vi "GenerateLog.vi"() -> (2 "JSON":string, 3 "MsgCluster":T1)   [LabVIEW 2020, in "ORM_Examples.lvlib" / "syslogs.lvclass"]
uses:
  syslogs.lvclass
  SysLogLog_cluster.ctl
  <vilib>/Utility/error.llb/DialogType.ctl
  <vilib>/numeric/Random Number (Range) U64.vi
  <vilib>/numeric/sub_Random U32.vi
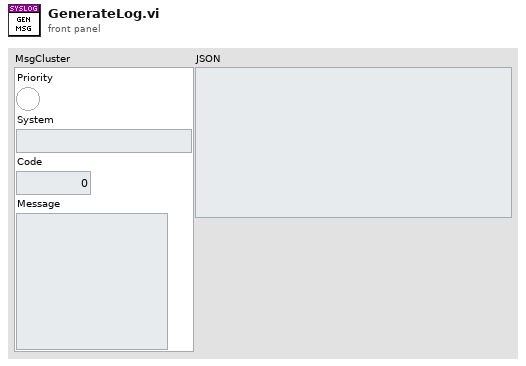
[diagram p1: front panel]
types:
  T1 = typedef "ORM_Examples.lvlib/syslogs.lvclass/SysLogLog_cluster.ctl" = cluster{"Priority":bool, "System":string, "Code":i32, "Message":string}
  T2 = typedef "DialogType.ctl" = u16
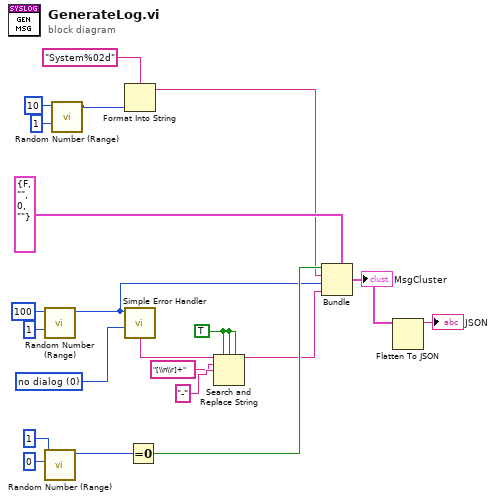
[diagram p0: block diagram]
diagram:
  w1 = TRUE ("ignore case? (F)")
  w19 = T2 0 items=["no dialog", "OK message", "continue or stop message", "OK message + warnings", "continue/stop + warnings"] ("type of dialog (OK msg:1)")
  n1 = call-poly <vilib>:"Random Number (Range).vi"("lower bound (0)"=u64 1, "upper bound (100)"=u64 100) -> ("number"=w8:u64)  [unwired: 9 in]
  n2 = call-poly <vilib>:"Random Number (Range).vi"("lower bound (0)"=u64 0, "upper bound (100)"=u64 1) -> ("number"=w15:u64)  [unwired: 9 in]
  n3 = call-poly <vilib>:"Random Number (Range).vi"("lower bound (0)"=u64 1, "upper bound (100)"=u64 10) -> ("number"=w11:u64)  [unwired: 9 in]
  n4 = Format Into String(format string="System%02d", w11) -> (resulting string=w9:string)  [unwired: 2 in, 1 out]
  n5 = call <vilib>:"Simple Error Handler.vi"("error code (no error:0)"=w8, "type of dialog (OK msg:1)"=w19) -> ("message"=w7:string)  [unwired: 3 in, 4 out]
  n6 = Equal To 0?(x=w15) -> (x = 0?=w14:bool)
  n7 = Search and Replace String(replace all?=w1, case sensitive?=w1, multiline?=w1, input string=w7, search string="[\\n\\r]+", replace string="-") -> (result string=w6:string)  [unwired: 2 in, 3 out]
  n8 = Bundle(cluster=T1 {"Priority"=FALSE, "System"="", "Code"=0, "Message"=""} ("Log"), "Priority"=w14, "System"=w9, "Code"=w8, "Message"=w6) -> (w5:T1)
  "MsgCluster" <- w5
  n9 = Flatten To JSON(anything=w5) -> (JSON string=→"JSON":string)  [unwired: 2 in, 1 out]
